vi "Simple Error Dialog.vi"(6 "Dialog Type":T1, 7 "Window Title":string, 11 "Error Interface in":refnum<class "Error Interface.lvclass">) -> (3 "User Action":T2)   [LabVIEW 2016, in "Stream Error.lvlib" / "Error Interface.lvclass"]
doc: "--\nCopyright © 2017 Composed SystemsI All rights reserved.\n\nAuthor: Jon McBee <jon.mcbee@composed.io>\n\nThis library is provided \"AS IS\" ,WITHOUT WARRANTIES OR\nCONDITIONS OF ANY KIND, either express or implied.\n\nComposed Systems -- composed.io\n\nStream 0.0.1.1\nJon McBee - Composed Systems\nCopyright (c) 2017, Composed Systems"
uses:
  <userlib>/Composed Systems/Stream/Error/Classes/Error Interface/Error Interface.lvclass
  <userlib>/Composed Systems/Stream/Error/Classes/Error Interface/User Actions.ctl
  <userlib>/Composed Systems/Stream/Error/Classes/Error Interface/Dialog Types.ctl
  <userlib>/Composed Systems/Stream/Error/Classes/Error Interface/Error Interface.lvclass/Error Interface.ctl
  <vilib>/Utility/miscctls.llb/LVRectTypeDef.ctl
panel:
  out "Long Call Chain:":string caption="Call Chain:"
  in  "Call Chain Visible":bool
  out "Short Call Chain:":string caption="Call Chain:"
  out "Error Source:":string
  out "Error Code:":string
  out "Error Scope:":string
  out "Possible Reason(s):":string
  in  "Continue":bool
  in  "Stop":bool
  in  "Abort":bool
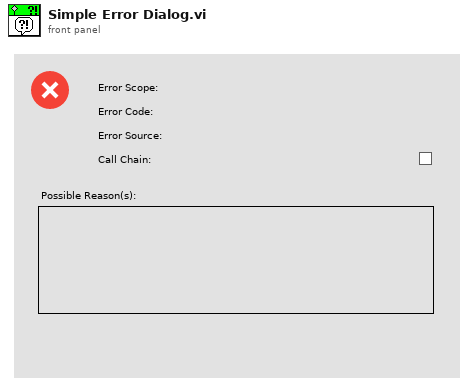
[diagram p1: front panel]
types:
  T1 = typedef "Stream Error.lvlib/Error Interface.lvclass/Dialog Types.ctl" = enum16{"No Dialog", "Continue Dialog", "Stop Dialog", "Abort Dialog"}
  T2 = typedef "Stream Error.lvlib/Error Interface.lvclass/User Actions.ctl" = enum16{"Continue", "Stop", "Abort"}
  T3 = typedef "LVRectTypeDef.ctl" = cluster{"Left":i16, "Top":i16, "Right":i16, "Bottom":i16}
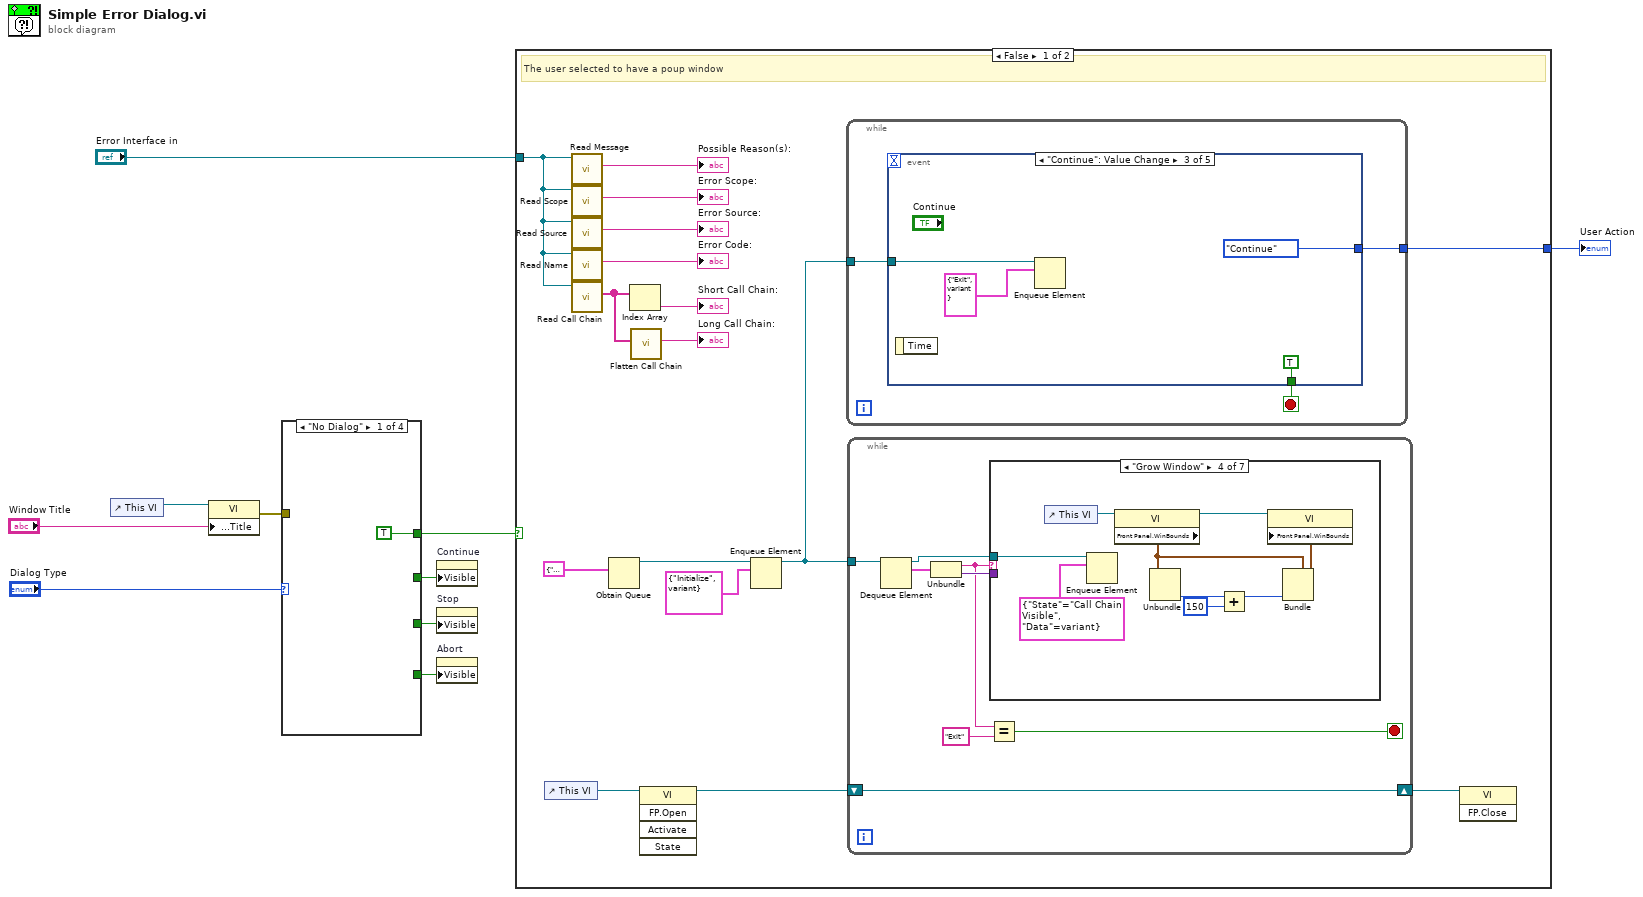
[diagram p0: block diagram]
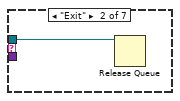
[diagram p3: hidden frame]
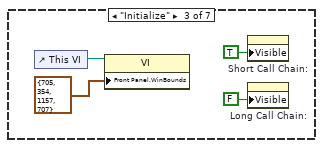
[diagram p4: hidden frame]
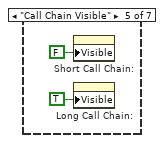
[diagram p5: hidden frame]
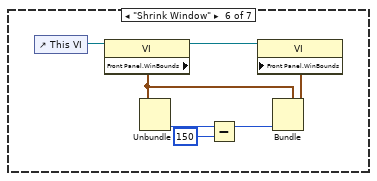
[diagram p6: hidden frame]
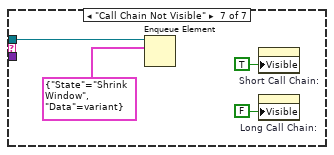
[diagram p7: hidden frame]
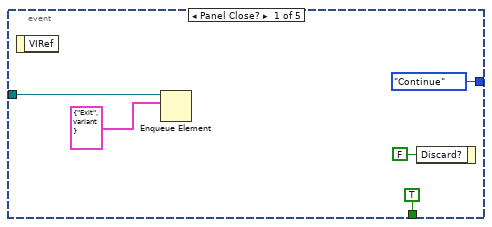
[diagram p8: hidden frame]
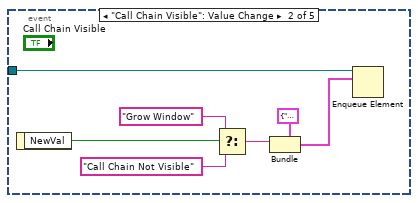
[diagram p9: hidden frame]
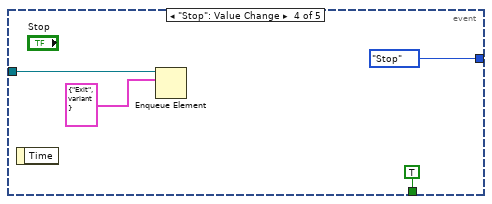
[diagram p10: hidden frame]
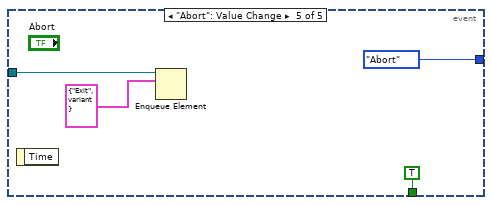
[diagram p11: hidden frame]
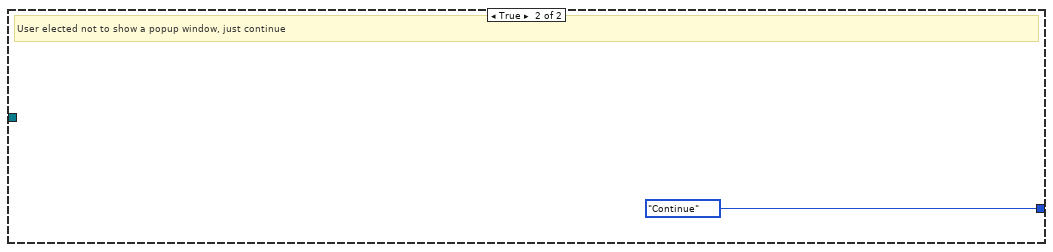
[diagram p12: hidden frame]
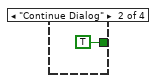
[diagram p13: hidden frame]
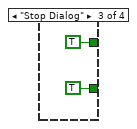
[diagram p14: hidden frame]
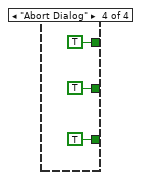
[diagram p15: hidden frame]
diagram:
  n1 = control-ref of="This VI"() -> (w10:refnum<vi>)
  n2 = property class="VI"(reference=w10, "Front Panel.Title"="Window Title") -> (error out=w5:errorcluster)  [unwired: 1 in, 1 out]
  n3 = case shown="\"No Dialog\"" "Dialog Type" {
    tunnel: [TRUE _ _ _] -> w7
    tunnel: w5 -> [_ _ _ _]
    tunnel: [_ TRUE TRUE TRUE] -> w4
    tunnel: [_ _ TRUE TRUE] -> w3
    tunnel: [_ _ _ TRUE] -> w2
    frame "No Dialog" {
    }
    frame "Continue Dialog" {
    }
    frame "Stop Dialog" {
    }
    frame "Abort Dialog" {
    }
  }
  n4 = property on="Continue" class="Bool"("Visible"=w4) -> ()  [unwired: 2 in, 2 out]
  n5 = property on="Stop" class="Bool"("Visible"=w3) -> ()  [unwired: 2 in, 2 out]
  n6 = property on="Abort" class="Bool"("Visible"=w2) -> ()  [unwired: 2 in, 2 out]
  n7 = case shown="False" w7 {
    tunnel: [w29 User_Actions."Continue" ("User Action")] -> w6
    tunnel: "Error Interface in" -> [w24 _]
    frame False {
      # "The user selected to have a poup window"
      n8 = control-ref of="This VI"() -> (w20:refnum<vi>)
      n9 = call <userlib>:"Read Message.vi"("Error Interface in"=w24) -> ("Message"=→"Possible Reason(s):":string)  [unwired: 8 in, 2 out]
      n10 = call <userlib>:"Read Scope.vi"("Error Interface in"=w24) -> ("Scope"=→"Error Scope:":string)  [unwired: 8 in, 2 out]
      n11 = call <userlib>:"Read Source.vi"("Error Interface in"=w24) -> ("Source"=→"Error Source:":string)  [unwired: 8 in, 2 out]
      n12 = call <userlib>:"Read Name.vi"("Error Interface in"=w24) -> ("Name"=→"Error Code:":string)  [unwired: 8 in, 2 out]
      n13 = call <userlib>:"Read Call Chain.vi"("Error Interface in"=w24) -> ("Call Chain"=w22:string[])  [unwired: 8 in, 2 out]
      n14 = Obtain Queue(element data type=cluster{"State":string, "Data":variant} {"State"="", "Data"=variant}) -> (queue out=w32:refnum<queue>)  [unwired: 4 in, 2 out]
      n15 = Index Array(array=w22) -> (element=→"Short Call Chain:":string)  [unwired: 1 in]
      n16 = call <userlib>:"Flatten Call Chain.vi"("Call Chain"=w22) -> ("Flattened Call Chain"=→"Long Call Chain:":string)  [unwired: 10 in]
      n17 = invoke class="VI" method="FP.Open"(reference=w20) -> (reference out=w19:refnum<vi>)  [unwired: 4 in, 4 out]
      n18 = Enqueue Element(queue=w32, element=cluster{"State":string, "Data":variant} {"State"="Initialize", "Data"=variant}) -> (queue out=w30:refnum<queue>)  [unwired: 2 in, 2 out]
      n19 = while {
        tunnel: w30 -> [w70]
        tunnel: [w69] -> w29
        stop <- w71 stop-if-true
        n20 = event shown="[2] \"Continue\": Value Change" {
          selector: _ -> [_ _ _ _ _]
          dyn-events: _ -> [_ _ _ _ _]
          timeout: _ -> [_ _ _ _ _]
          tunnel: [TRUE ("Discard?") _ TRUE ("Discard?") TRUE ("Discard?") TRUE ("Discard?")] -> w71
          tunnel: w70 -> [w75 w83 w86 w90 w94]
          tunnel: [User_Actions."Continue" ("User Action") _ User_Actions."Continue" ("User Action") User_Actions."Stop" ("User Action") User_Actions."Abort" ("User Action")] -> w69
          event Panel Close? {
            n21 = event-data() -> ()  [unwired: 1 in, 1 out]
            n22 = Enqueue Element(queue=w75, element=cluster{"State":string, "Data":variant} {"State"="Exit", "Data"=variant}) -> ()  [unwired: 2 in, 3 out]
            n23 = event-data("Discard?"=FALSE) -> ()  [unwired: 1 in, 1 out]
          }
          event "Call Chain Visible": Value Change {
            n24 = event-data() -> ("NewVal"=w80:bool)  [unwired: 1 in]
            n25 = Select(t="Grow Window" ("State"), s=w80, f="Call Chain Not Visible" ("State")) -> (s? t:f=w78:string)
            n26 = Bundle(cluster=cluster{"State":string, "Data":variant} {"State"="", "Data"=variant} ("element"), "State"=w78) -> (w81:cluster{"State":string, "Data":variant})  [unwired: 1 in]
            n27 = Enqueue Element(queue=w83, element=w81) -> ()  [unwired: 2 in, 3 out]
          }
          event "Continue": Value Change {
            n28 = event-data() -> ()  [unwired: 1 in, 1 out]
            n29 = Enqueue Element(queue=w86, element=cluster{"State":string, "Data":variant} {"State"="Exit", "Data"=variant}) -> ()  [unwired: 2 in, 3 out]
          }
          event "Stop": Value Change {
            n30 = event-data() -> ()  [unwired: 1 in, 1 out]
            n31 = Enqueue Element(queue=w90, element=cluster{"State":string, "Data":variant} {"State"="Exit", "Data"=variant}) -> ()  [unwired: 2 in, 3 out]
          }
          event "Abort": Value Change {
            n32 = event-data() -> ()  [unwired: 1 in, 1 out]
            n33 = Enqueue Element(queue=w94, element=cluster{"State":string, "Data":variant} {"State"="Exit", "Data"=variant}) -> ()  [unwired: 2 in, 3 out]
          }
        }
      }
      n34 = while {
        tunnel: w30 -> [w41]
        shift-right: [w34] -> w18
        shift-left: w19 -> [w34]
        stop <- w36 stop-if-true
        n35 = Dequeue Element(queue=w41) -> (queue out=w35:refnum<queue>, element=w40:cluster{"State":string, "Data":variant})  [unwired: 2 in, 2 out]
        n36 = Unbundle(w40) -> ("State"=w38:string, "Data"=w39:variant)
        n37 = Equal?(x=w38, y="Exit") -> (x = y?=w36:bool)
        n38 = case shown="\"Grow Window\"" w38 {
          tunnel: w39 -> [_ _ _ _ _ _ _]
          tunnel: w35 -> [_ w42 _ w48 _ _ w65]
          frame Default {
          }
          frame "Exit" {
            n39 = Release Queue(queue=w42) -> ()  [unwired: 2 in, 3 out]
          }
          frame "Initialize" {
            n40 = control-ref of="This VI"() -> (w44:refnum<vi>)
            n41 = property class="VI"(reference=w44, "Front Panel.WinBounds"=T3 {"Left"=705, "Top"=354, "Right"=1157, "Bottom"=707} ("Front Panel Window:Window Bounds")) -> ()  [unwired: 1 in, 2 out]
            n42 = property on="Short Call Chain:" class="Str"("Visible"=TRUE) -> ()  [unwired: 2 in, 2 out]
            n43 = property on="Long Call Chain:" class="Str"("Visible"=FALSE) -> ()  [unwired: 2 in, 2 out]
          }
          frame "Grow Window" {
            n44 = control-ref of="This VI"() -> (w55:refnum<vi>)
            n45 = Enqueue Element(queue=w48, element=cluster{"State":string, "Data":variant} {"State"="Call Chain Visible", "Data"=variant}) -> ()  [unwired: 2 in, 3 out]
            n46 = property class="VI"(reference=w55) -> (reference out=w54:refnum<vi>, "Front Panel.WinBounds"=w53:T3)  [unwired: 1 in, 1 out]
            n47 = Unbundle(w53) -> ("Bottom"=w52:i16)  [unwired: 3 out]
            n48 = Add(x=w52, y=i16 150) -> (x+y=w50:i16)
            n49 = Bundle(cluster=w53, "Bottom"=w50) -> (w51:T3)  [unwired: 3 in]
            n50 = property class="VI"(reference=w54, "Front Panel.WinBounds"=w51) -> ()  [unwired: 1 in, 2 out]
          }
          frame "Call Chain Visible" {
            n51 = property on="Short Call Chain:" class="Str"("Visible"=FALSE) -> ()  [unwired: 2 in, 2 out]
            n52 = property on="Long Call Chain:" class="Str"("Visible"=TRUE) -> ()  [unwired: 2 in, 2 out]
          }
          frame "Shrink Window" {
            n53 = control-ref of="This VI"() -> (w64:refnum<vi>)
            n54 = property class="VI"(reference=w64) -> (reference out=w63:refnum<vi>, "Front Panel.WinBounds"=w62:T3)  [unwired: 1 in, 1 out]
            n55 = Unbundle(w62) -> ("Bottom"=w61:i16)  [unwired: 3 out]
            n56 = Subtract(x=w61, y=i16 150) -> (x-y=w59:i16)
            n57 = Bundle(cluster=w62, "Bottom"=w59) -> (w60:T3)  [unwired: 3 in]
            n58 = property class="VI"(reference=w63, "Front Panel.WinBounds"=w60) -> ()  [unwired: 1 in, 2 out]
          }
          frame "Call Chain Not Visible" {
            n59 = Enqueue Element(queue=w65, element=cluster{"State":string, "Data":variant} {"State"="Shrink Window", "Data"=variant}) -> ()  [unwired: 2 in, 3 out]
            n60 = property on="Short Call Chain:" class="Str"("Visible"=TRUE) -> ()  [unwired: 2 in, 2 out]
            n61 = property on="Long Call Chain:" class="Str"("Visible"=FALSE) -> ()  [unwired: 2 in, 2 out]
          }
        }
      }
      n62 = invoke class="VI" method="FP.Close"(reference=w18) -> ()  [unwired: 2 in, 3 out]
    }
    frame True {
      # "User elected not to show a popup window, just continue"
    }
  }
  "User Action" <- w6
